vi "Initial Control Write.vi"(8 "error in":errorcluster, 10 "Controlword":T3, 11 "IgusMotorDrive in":refnum<class "IgusMotorDrive.lvclass">) -> (0 "error out":errorcluster, 1 "Response":T1={"Function Code"=1, "Data"=[], "RTU_DataBytes"=0} {"Data" format="%.0x"}, 2 "Command":T1={"Function Code"=1, "Data"=[], "RTU_DataBytes"=0} {"Data" format="%.0x"}, 3 "IgusMotorDrive out":refnum<class "IgusMotorDrive.lvclass">, 5 "Controlword Out":T2)   [LabVIEW 2016, in "IgusMotorDrive.lvclass"]
doc: "Writes the control command to the drive\n\n<b>Copyright (C) 2018 Control Software Solutions Limited. All rights reserved. </b>"
uses:
  IgusMotorDrive.lvclass
  typedefs/Controlword--enum.ctl
  typedefs/Controlword--cluster.ctl
  Libraries/Modbus-Master/MB_PDU/MB_PDU_Cluster.ctl
  IgusMotorDrive.lvclass/IgusMotorDrive.ctl
  Libraries/Modbus-Master/MB_Master_TCP/MB_Master_TCP.lvclass
  C:/Projekte/Lufft/CHM8K/igus Stages/igusPositioningSystem/Modules/Libraries/Modbus-Master/MB_Master/MB_Master.lvclass
  Libraries/Modbus-Master/MB Master.lvlib
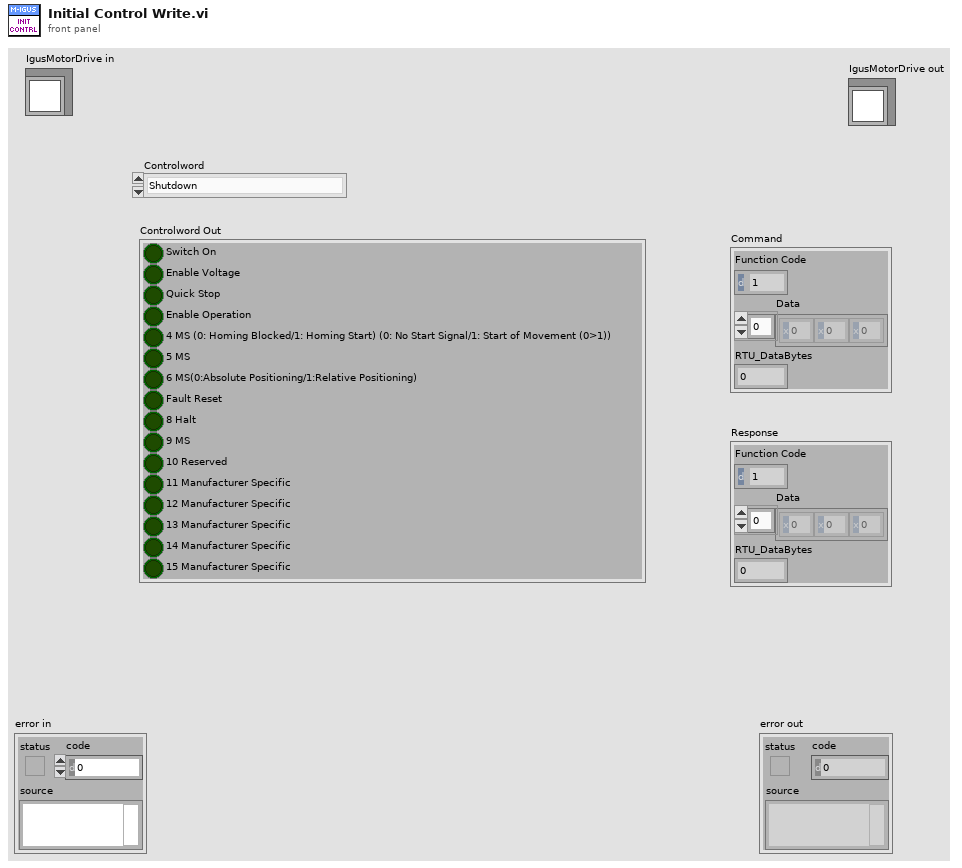
[diagram p1: front panel]
types:
  T1 = typedef "MB Master.lvlib/MB_PDU_Cluster.ctl" = cluster{"Function Code":u8, "Data":u8[], "RTU_DataBytes":i32}
  T2 = typedef "IgusMotorDrive.lvclass/Controlword--cluster.ctl" = cluster{"Switch On":bool, "Enable Voltage":bool, "Quick Stop":bool, "Enable Operation":bool, "4 MS (0: Homing Blocked/1: Homing Start) (0: No Start Signal/1: Start of Movement (0>1))":bool, "5 MS":bool, "6 MS(0:Absolute Positioning/1:Relative Positioning)":bool, "Fault Reset":bool, "8 Halt":bool, "9 MS":bool, "10 Reserved":bool, "11 Manufacturer Specific":bool, "12 Manufacturer Specific":bool, "13 Manufacturer Specific":bool, "14 Manufacturer Specific":bool, "15 Manufacturer Specific":bool}
  T3 = typedef "IgusMotorDrive.lvclass/Controlword--enum.ctl" = enum16{"Shutdown", "Switch On", "Switch On and Enable Operation", "Disable Voltage", "Halt", "Quick Stop", "Disable Operation", "Enable Operation", "Fault Reset"}
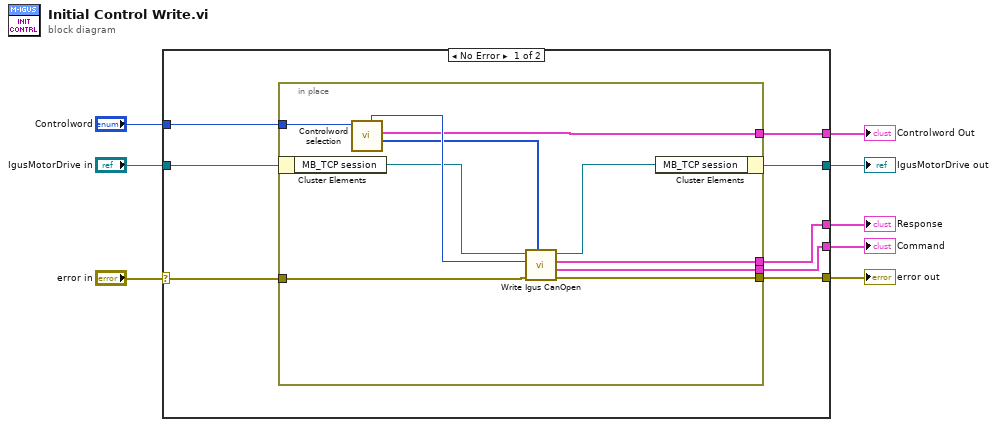
[diagram p0: block diagram]
diagram:
  n1 = case shown="No Error" "error in" {
    selector: "error in" -> [w16 w28]
    tunnel: [w15 w28] -> w7
    tunnel: [w9 w27] -> w5
    tunnel: "IgusMotorDrive in" -> [w11 w27]
    tunnel: [w14 _] -> w4
    tunnel: [w13 _] -> w3
    tunnel: [w12 _] -> w2
    tunnel: "Controlword" -> [w10 _]
    frame No Error {
      n2 = in-place {
        in-place-border: w16 -> [w25]
        in-place-border: [w24] -> w15
        in-place-border: [w23] -> w14
        in-place-border: [w22] -> w13
        in-place-border: [w21] -> w12
        in-place-border: w10 -> [w17]
        n3 = in-place-cluster #1(w11) -> ("MB_TCP session"=w19:refnum<class "MB_Master_TCP.lvclass">)
        n4 = call "Controlword selection.vi"("Controlword"=w17) -> ("Control Word Data"=w20:u8[], "Controlword Out"=w23:T2, "address"=w26:u16)  [unwired: 7 in, 1 out]
        n5 = call "Write Igus CanOpen.vi"("Data [1-4]"=w20, "error in (no error)"=w25, "Address"=w26, "MB session in"=w19) -> ("error out"=w24:errorcluster, "Command"=w22:T1, "Response"=w21:T1, "MB session out"=w18:refnum<class "MB_Master_TCP.lvclass">)  [unwired: 4 in]
        n6 = in-place-cluster #1("MB_TCP session"=w18) -> (w9:refnum<class "IgusMotorDrive.lvclass">)
      }
    }
    frame Error {
    }
  }
  "error out" <- w7
  "IgusMotorDrive out" <- w5
  "Controlword Out" <- w4
  "Command" <- w3
  "Response" <- w2
